vi "Draw History.vi"(8 "error in (no error)":errorcluster, 11 "StatusHistory in":refnum<class "StatusHistory.lvclass">) -> (0 "error out":errorcluster, 3 "StatusHistory out":refnum<class "StatusHistory.lvclass">)   [LabVIEW 2020, in "StatusHistory.lvclass"]
doc: "<b> </b> <b> </b>\n©2016 Q Software Innovations, LLC (QSI)\nwritten by Quentin Alldredge\nproduced in LabVIEW 2015\n\nsupport@qsoftwareinnovations.com\nwww.qsoftwareinnovations.com\n\nAll rights reserved.\n\nRedistribution and use in source and binary forms, with or without modification, are permitted provided that the following conditions are met:\n\n * Redistributions of source code must retain the above copyright notice, this list of conditions and the following disclaimer.\n * Redistributions in binary form must reproduce the above copyright notice, this list of conditions and the following disclaimer in the documentation and/or other materials provided with the distribution.\n * Neither the name of Q Software Innovations, LLC. nor the names of its contributors may be used to endorse or promote products derived from this software without specific prior written permission.\n\nTHIS SOFTWARE IS PROVIDED BY THE COPYRIGHT HOLDERS AND CONTRIBUTORS \"AS IS\" AND ANY EXPRESS OR IMPLIED WARRANTIES, INCLUDING, BUT NOT LIMITED TO, THE IMPLIED WARRANTIES OF MERCHANTABILITY AND FITNESS FOR A PARTICULAR PURPOSE ARE DISCLAIMED. IN NO EVENT SHALL THE COPYRIGHT OWNER OR CONTRIBUTORS BE LIABLE FOR ANY DIRECT, INDIRECT, INCIDENTAL, SPECIAL, EXEMPLARY, OR CONSEQUENTIAL DAMAGES (INCLUDING, BUT NOT LIMITED TO, PROCUREMENT OF SUBSTITUTE GOODS OR SERVICES; LOSS OF USE, DATA, OR PROFITS; OR BUSINESS INTERRUPTION) HOWEVER CAUSED AND ON ANY THEORY OF LIABILITY, WHETHER IN CONTRACT, STRICT LIABILITY, OR TORT (INCLUDING NEGLIGENCE OR OTHERWISE) ARISING IN ANY WAY OUT OF THE USE OF THIS SOFTWARE, EVEN IF ADVISED OF THE POSSIBILITY OF SUCH DAMAGE."
uses:
  StatusHistory.lvclass
  StatusHistory.lvclass/StatusHistory.ctl
  Read History Size.vi
  Read Direction.vi
  Read Most Recent Color.vi
  Read Least Recent Color.vi
  Read Lock Scrolling.vi
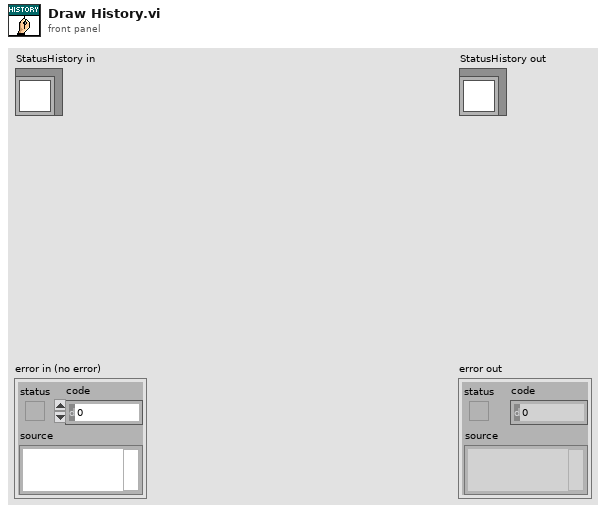
[diagram p1: front panel]
types:
  T1 = typedef "StatusHistory.lvclass/Direction.ctl" = enum16{"Descending", "Ascending"}
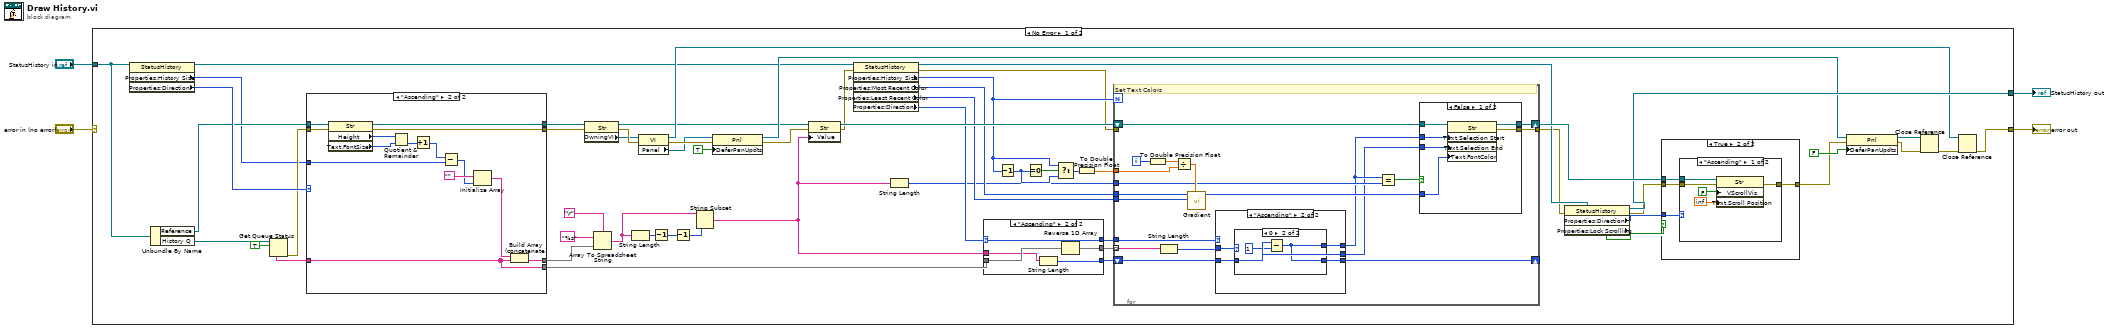
[diagram p0: block diagram]
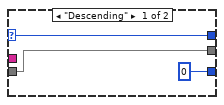
[diagram p2: hidden frame]
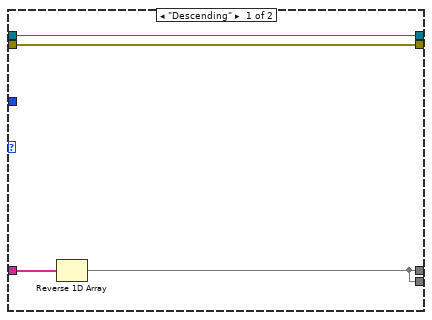
[diagram p3: hidden frame]
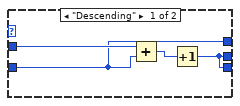
[diagram p5: hidden frame]
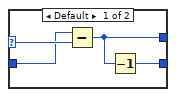
[diagram p6: hidden frame]
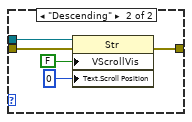
[diagram p8: hidden frame]
diagram:
  n1 = case shown="No Error" "error in (no error)" {
    selector: "error in (no error)" -> [_ w145]
    tunnel: [w37 w145] -> w3
    tunnel: [w48 w144] -> w1
    tunnel: "StatusHistory in" -> [w49 w144]
    frame No Error {
      n2 = property class="StatusHistory"(reference=w49) -> (reference out=w23:refnum<class "StatusHistory.lvclass">, "Properties:History Size"=w21:u32, "Properties:Direction"=w35:T1)  [unwired: 1 in, 1 out]
      n3 = Unbundle By Name(w49) -> ("Reference"=w33:refnum<vi>, "History Q"=w60:refnum<queue>)
      n4 = Get Queue Status(queue=w60, return elements? (F)=TRUE) -> (error out=w31:errorcluster, elements=w47:string[])  [unwired: 1 in, 6 out]
      n5 = case shown="\"Ascending\"" w35 {
        tunnel: w47 -> [w73 w74]
        tunnel: [w70 w79] -> w5
        tunnel: w33 -> [w72 w87]
        tunnel: [w72 w83] -> w32
        tunnel: w31 -> [w71 w86]
        tunnel: [w71 w82] -> w30
        tunnel: w21 -> [_ w77]
        tunnel: [w70 w74] -> w6
        frame "Descending" {
          n6 = Reverse 1D Array(array=w73) -> (reversed array=w70:string[])
        }
        frame "Ascending" {
          n7 = property class="Str"(reference=w87, error in=w86) -> (reference out=w83:refnum<vi>, error out=w82:errorcluster, "Height"=w85:u32, "Text.FontSize"=w84:u32)
          n8 = Quotient & Remainder(x=w85, y=w84) -> (floor(x/y)=w81:u32)  [unwired: 1 out]
          n9 = Increment(x=w81) -> (x+1=w78:u32)
          n10 = Subtract(x=w78, y=w77) -> (x-y=w75:u32)
          n11 = Initialize Array("", w75) -> (w80:string[])
          n12 = Build Array (concatenate)(w80, w74) -> (w79:string[])
        }
      }
      n13 = property class="Str"(reference=w32, error in=w30) -> (reference out=w29:refnum<vi>, error out=w57:errorcluster, "OwningVI"=w45:refnum<vi>)
      n14 = Array To Spreadsheet String(delimiter (Tab)="\r", array=w5, 3:"%s" ("format string")) -> (spreadsheet string=w55:string)
      n15 = String Length(string=w55) -> (length=w54:i32)
      n16 = property class="VI"(reference=w45, error in=w57) -> (reference out=w36:refnum<vi>, error out=w46:errorcluster, "Panel"=w44:refnum<vi>)
      n17 = Decrement(x=w54) -> (x-1=w53:i32)
      n18 = Decrement(x=w53) -> (x-1=w52:i32)
      n19 = String Subset(string=w55, length (rest)=w52) -> (substring=w8:string)  [unwired: 1 in]
      n20 = property class="Pnl"(reference=w44, error in=w46, "DeferPanUpdts"=TRUE ("Defer Panel Updates")) -> (reference out=w40:refnum<vi>, error out=w28:errorcluster)
      n21 = property class="Str"(reference=w29, error in=w28, "Value"=w8) -> (reference out=w27:refnum<vi>, error out=w19:errorcluster)
      n22 = property class="StatusHistory"(reference=w23, error in=w19) -> (reference out=w22:refnum<class "StatusHistory.lvclass">, error out=w18:errorcluster, "Properties:History Size"=w20:u32, "Properties:Most Recent Color"=w17:u32, "Properties:Least Recent Color"=w16:u32, "Properties:Direction"=w15:T1)
      n23 = String Length(string=w8) -> (length=w7:i32)
      n24 = case shown="\"Ascending\"" w15 {
        selector: w15 -> [w63 w69]
        tunnel: w6 -> [w62 w68]
        tunnel: [0 w66] -> w14
        tunnel: [w63 w69] -> w13
        tunnel: [w62 w65] -> w9
        tunnel: w8 -> [_ w67]
        frame "Descending" {
        }
        frame "Ascending" {
          n25 = String Length(string=w67) -> (length=w66:i32)
          n26 = Reverse 1D Array(array=w68) -> (reversed array=w65:string[])
        }
      }
      n27 = Decrement(x=w20) -> (x-1=w25:u32)
      n28 = Equal To 0?(x=w25) -> (x = 0?=w26:bool)
      n29 = Select(t=w20, s=w26, f=w25) -> (s? t:f=w24:u32)
      n30 = To Double Precision Float(number=w24) -> (double precision float=w34:dbl)
      n31 = for {
        N: w20 -> [_]
        tunnel: w34 -> [w105]
        tunnel: w18 -> [_]
        tunnel: [w102] -> w11
        shift-right: [w101] -> w56
        shift-left: w27 -> [w100]
        tunnel: w17 -> [w99]
        tunnel: w16 -> [w98]
        tunnel: w13 -> [w97]
        shift-right: [w88] -> _
        shift-left: w14 -> [w91]
        tunnel: w9 -> [w95] mode=indexing
        tunnel: w7 -> [w92]
        i -> [w96]
        # "Set Text Colors"
        n32 = To Double Precision Float(number=w96) -> (double precision float=w106:dbl)
        n33 = String Length(string=w95) -> (length=w94:i32)
        n34 = Divide(x=w106, y=w105) -> (x/y=w104:dbl)
        n35 = call "Gradient.vi"("Percent"=w104, "End Color"=w98, "Start Color"=w99) -> ("Gradient Color"=w103:u32)  [unwired: 8 in]
        n36 = case shown="\"Ascending\"" w97 {
          tunnel: w91 -> [w115 w120]
          tunnel: [w114 w120] -> w89
          tunnel: w94 -> [w116 w121]
          tunnel: [w115 w118] -> w90
          tunnel: [w114 w119] -> w88
          frame "Descending" {
            n37 = Add(x=w116, y=w115) -> (x+y=w117:i32)
            n38 = Increment(x=w117) -> (x+1=w114:i32)
          }
          frame "Ascending" {
            n39 = case shown="0" w121 {
              selector: w121 -> [w125 _]
              tunnel: w120 -> [w124 w128]
              tunnel: [w123 w126] -> w119
              tunnel: [w122 w126] -> w118
              frame Default {
                n40 = Subtract(x=w124, y=w125) -> (x-y=w122:i32)
                n41 = Decrement(x=w122) -> (x-1=w123:i32)
              }
              frame 0 {
                n42 = Subtract(x=w128, y=1) -> (x-y=w126:i32)
              }
            }
          }
        }
        n43 = Equal?(x=w90, y=w92) -> (x = y?=w93:bool)
        n44 = case shown="False" w93 {
          tunnel: w103 -> [w112 _]
          tunnel: [w111 _] -> w102
          tunnel: [w110 w113] -> w101
          tunnel: w100 -> [w109 w113]
          tunnel: w90 -> [w108 _]
          tunnel: w89 -> [w107 _]
          frame False {
            n45 = property class="Str"(reference=w109, "Text.Selection Start"=w108, "Text.Selection End"=w107, "Text.FontColor"=w112) -> (reference out=w110:refnum<vi>, error out=w111:errorcluster)  [unwired: 1 in]
          }
          frame True {
          }
        }
      }
      n46 = property class="StatusHistory"(reference=w22, error in=w11) -> (reference out=w48:refnum<class "StatusHistory.lvclass">, error out=w10:errorcluster, "Properties:Direction"=w51:T1, "Properties:Lock Scrolling"=w50:bool)
      n47 = case shown="True" w50 {
        tunnel: w56 -> [_ w133]
        tunnel: w10 -> [w129 w132]
        tunnel: w51 -> [_ w131]
        tunnel: [w129 w130] -> w12
        frame False {
        }
        frame True {
          n48 = case shown="\"Ascending\"" w131 {
            tunnel: w133 -> [w138 w143]
            tunnel: w132 -> [w137 w142]
            tunnel: [w134 w139] -> w130
            frame "Ascending" {
              n49 = property class="Str"(reference=w138, error in=w137, "VScrollVis"=FALSE ("Vertical Scrollbar Visible"), "Text.Scroll Position"=inf) -> (error out=w134:errorcluster)  [unwired: 1 out]
            }
            frame "Descending" {
              n50 = property class="Str"(reference=w143, error in=w142, "VScrollVis"=FALSE ("Vertical Scrollbar Visible"), "Text.Scroll Position"=u32 0) -> (error out=w139:errorcluster)  [unwired: 1 out]
            }
          }
        }
      }
      n51 = property class="Pnl"(reference=w40, error in=w12, "DeferPanUpdts"=FALSE ("Defer Panel Updates")) -> (reference out=w39:refnum<vi>, error out=w41:errorcluster)
      n52 = Close Reference(reference=w39, error in (no error)=w41) -> (error out=w38:errorcluster)
      n53 = Close Reference(reference=w36, error in (no error)=w38) -> (error out=w37:errorcluster)
    }
    frame Error {
    }
  }
  "error out" <- w3
  "StatusHistory out" <- w1
